vi "SaveExperiment.vi"(8 "Error In":errorcluster, 11 "Experiment":T1={"File Path"=path "", "Operator"="Operator", "Project"="Project Description", "Target Dose (dpa)"=0.0, "Sample"={"Name"="", "Description"="", "Molar Mass (g/mol)"=0.0, "Density (g/cm^3)"=0.0, "Irradiation Area (cm^2)"=0.0, "SRIM Damage Peak (disp * ions/cm)"=0.0}, "Beam Line"={"Type"=enum."Ion Beam Analysis", "Ion"=enum."H", "Charge State"=0, "Total Source Ion Energy (kV)"=nan}, "Runs"=[]} {"Beam Line"."Charge State" min=1}) -> (0 "Error Out":errorcluster)   [LabVIEW 2012]
uses:
  Experiment.ctl
  Sample.ctl
  BeamLine.ctl
  BeamLineType.ctl
  BeamLineIon.ctl
  ExperimentRun.ctl
  ExperimentRunTiming.ctl
  ExperimentRunDose.ctl
  ExperimentRunFluence.ctl
  ExperimentRunTotalCharge.ctl
  <vilib>/xml/Close Reference(Node).vi
  <vilib>/xml/NI_XML.lvlib
  <resource>/objmgr/DOMUserDefRef.rc
panel:
  out "XML":string
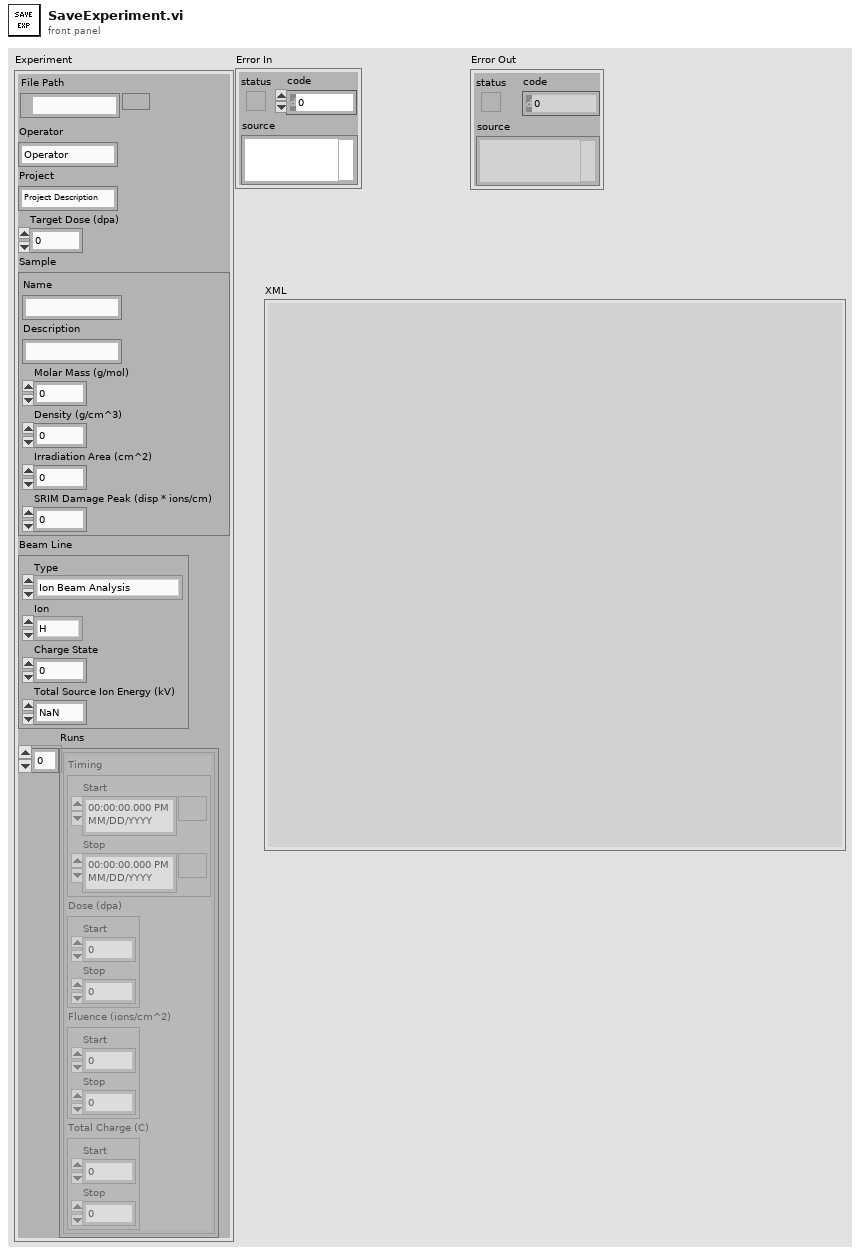
[diagram p1: front panel]
types:
  T1 = typedef "Experiment.ctl" = cluster{"File Path":path, "Operator":string, "Project":string, "Target Dose (dpa)":dbl, "Sample":T2, "Beam Line":T3, "Runs":T6[]}
  T2 = typedef "Sample.ctl" = cluster{"Name":string, "Description":string, "Molar Mass (g/mol)":dbl, "Density (g/cm^3)":dbl, "Irradiation Area (cm^2)":dbl, "SRIM Damage Peak (disp * ions/cm)":dbl}
  T3 = typedef "BeamLine.ctl" = cluster{"Type":T4, "Ion":T5, "Charge State":u8, "Total Source Ion Energy (kV)":dbl}
  T4 = typedef "BeamLineType.ctl" = enum16{"Ion Beam Analysis", "Auxiliary", "Radiation Damage"}
  T5 = typedef "BeamLineIon.ctl" = enum16{"H", "He", "C", "Fe", "Ni", "Pt", "Si", "Ag", "Au"}
  T6 = typedef "ExperimentRun.ctl" = cluster{"Timing":T7, "Dose (dpa)":T8, "Fluence (ions/cm^2)":T9, "Total Charge (C)":T10}
  T7 = typedef "ExperimentRunTiming.ctl" = cluster{"Start":timestamp, "Stop":timestamp}
  T8 = typedef "ExperimentRunDose.ctl" = cluster{"Start":dbl, "Stop":dbl}
  T9 = typedef "ExperimentRunFluence.ctl" = cluster{"Start":dbl, "Stop":dbl}
  T10 = typedef "ExperimentRunTotalCharge.ctl" = cluster{"Start":dbl, "Stop":dbl}
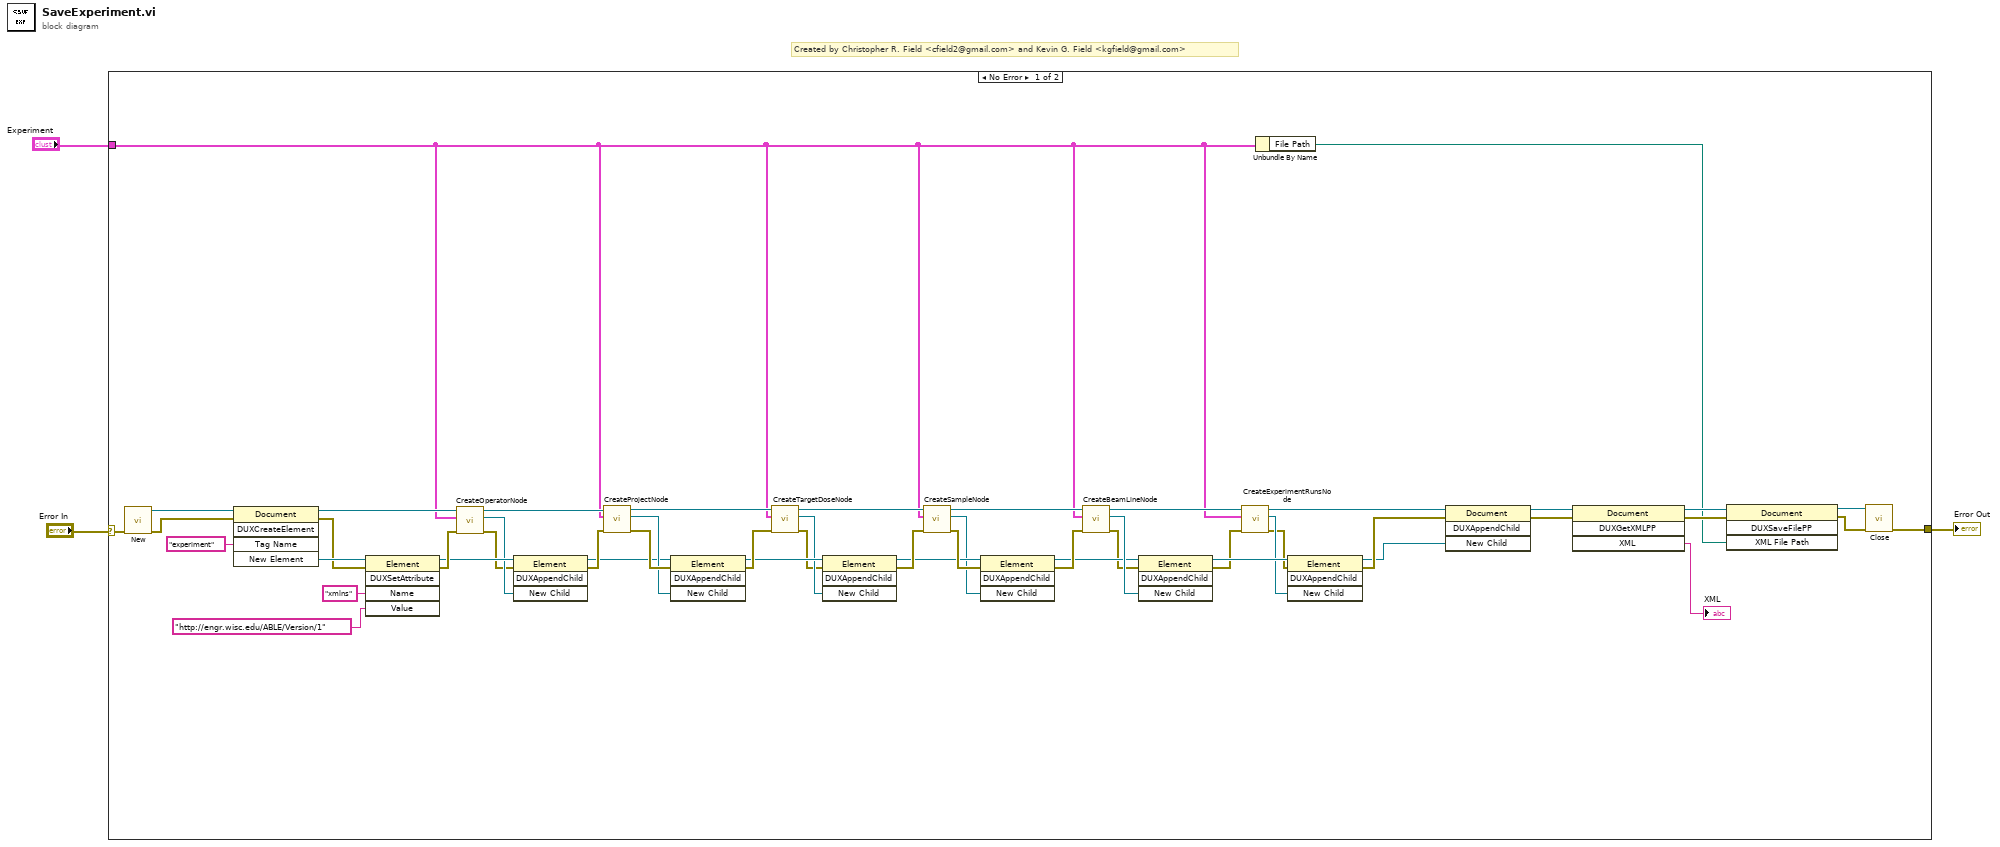
[diagram p0: block diagram]
diagram:
  # "Created by Christopher R. Field <cfield2@gmail.com> and Kevin G. Field <kgfield@gmail.com>"
  n1 = case shown="No Error" "Error In" {
    selector: "Error In" -> [w54 w55]
    tunnel: "Experiment" -> [w16 _]
    tunnel: [w10 w55] -> w2
    frame No Error {
      n2 = call <vilib>:"New.vi"("error in (no error)"=w54) -> ("error out"=w27:errorcluster, "DOM document out"=w53:refnum<k20>)  [unwired: 7 in]
      n3 = invoke class="Document" method="DUXCreateElement"(reference=w53, error in=w27, "Tag Name"="experiment") -> (reference out=w47:refnum<k20>, error out=w50:errorcluster, "New Element"=w51:refnum<k20>)  [unwired: 2 in, 2 out]
      n4 = invoke class="Element" method="DUXSetAttribute"(reference=w51, error in=w50, "Name"="xmlns", "Value"="http://engr.wisc.edu/ABLE/Version/1") -> (reference out=w45:refnum<k20>, error out=w46:errorcluster)  [unwired: 1 in, 3 out]
      n5 = call "CreateOperatorNode.vi"("Error In"=w46, "Experiment"=w16, "DOM Document In"=w47) -> ("Error out"=w43:errorcluster, "Operator Node"=w44:refnum<k20>, "DOM Document Out"=w41:refnum<k20>)  [unwired: 6 in]
      n6 = invoke class="Element" method="DUXAppendChild"(reference=w45, error in=w43, "New Child"=w44) -> (reference out=w38:refnum<k20>, error out=w42:errorcluster)  [unwired: 1 in, 2 out]
      n7 = call "CreateProjectNode.vi"("Error In"=w42, "Experiment"=w16, "DOM Document In"=w41) -> ("Error out"=w40:errorcluster, "Project Node"=w39:refnum<k20>, "DOM Document Out"=w37:refnum<k20>)  [unwired: 6 in]
      n8 = invoke class="Element" method="DUXAppendChild"(reference=w38, error in=w40, "New Child"=w39) -> (reference out=w35:refnum<k20>, error out=w36:errorcluster)  [unwired: 1 in, 2 out]
      n9 = call "CreateTargetDoseNode.vi"("Error In"=w36, "Experiment"=w16, "DOM Document In"=w37) -> ("Error out"=w33:errorcluster, "Target Dose Node"=w34:refnum<k20>, "DOM Document Out"=w32:refnum<k20>)  [unwired: 6 in]
      n10 = invoke class="Element" method="DUXAppendChild"(reference=w35, error in=w33, "New Child"=w34) -> (reference out=w29:refnum<k20>, error out=w31:errorcluster)  [unwired: 1 in, 2 out]
      n11 = call "CreateSampleNode.vi"("Error In"=w31, "Experiment"=w16, "DOM Document In"=w32) -> ("Error out"=w30:errorcluster, "Sample Node"=w28:refnum<k20>, "DOM Document Out"=w26:refnum<k20>)  [unwired: 6 in]
      n12 = invoke class="Element" method="DUXAppendChild"(reference=w29, error in=w30, "New Child"=w28) -> (reference out=w23:refnum<k20>, error out=w25:errorcluster)  [unwired: 1 in, 2 out]
      n13 = call "CreateBeamLineNode.vi"("Error In"=w25, "Experiment"=w16, "DOM Document In"=w26) -> ("Error out"=w22:errorcluster, "Beam Line Node"=w24:refnum<k20>, "DOM Document Out"=w21:refnum<k20>)  [unwired: 6 in]
      n14 = invoke class="Element" method="DUXAppendChild"(reference=w23, error in=w22, "New Child"=w24) -> (reference out=w20:refnum<k20>, error out=w18:errorcluster)  [unwired: 1 in, 2 out]
      n15 = call "CreateExperimentRunsNode.vi"("Error In"=w18, "Experiment"=w16, "DOM Document In"=w21) -> ("Error out"=w17:errorcluster, "Experiment Runs Node"=w19:refnum<k20>, "DOM Document Out"=w8:refnum<k20>)  [unwired: 6 in]
      n16 = Unbundle By Name(w16) -> ("File Path"=w13:path)
      n17 = invoke class="Element" method="DUXAppendChild"(reference=w20, error in=w17, "New Child"=w19) -> (reference out=w6:refnum<k20>, error out=w7:errorcluster)  [unwired: 1 in, 2 out]
      n18 = invoke class="Document" method="DUXAppendChild"(reference=w8, error in=w7, "New Child"=w6) -> (reference out=w5:refnum<k20>, error out=w4:errorcluster)  [unwired: 1 in, 2 out]
      n19 = invoke class="Document" method="DUXGetXMLPP"(reference=w5, error in=w4) -> (reference out=w15:refnum<k20>, error out=w14:errorcluster, "XML"=→"XML":string)  [unwired: 2 in, 1 out]
      n20 = invoke class="Document" method="DUXSaveFilePP"(reference=w15, error in=w14, "XML File Path"=w13) -> (reference out=w12:refnum<k20>, error out=w11:errorcluster)  [unwired: 1 in, 2 out]
      n21 = call-poly <vilib>:"Close.vi"("error in (no error)"=w11, "node"=w12) -> ("error out"=w10:errorcluster)  [unwired: 7 in]
    }
    frame Error {
    }
  }
  "Error Out" <- w2
